vi "_RT_CtrlLoop_ExperimentCondition.vi"(6 "NewExpVar.lvclass":refnum<class "ExpVar.lvclass">, 8 "error in":errorcluster) -> (0 "error out":errorcluster)   [LabVIEW 2018]
uses:
  PublicSubVI/NewExpVar/ExpVar.lvclass
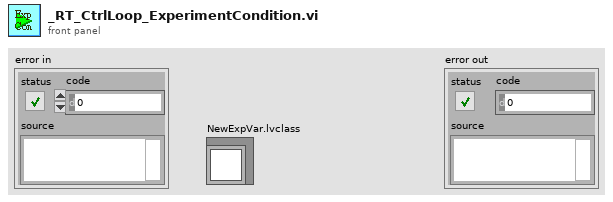
[diagram p1: front panel]
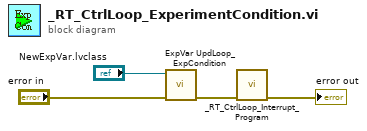
[diagram p0: block diagram]
diagram:
  n1 = call-dynamic "ExpVar UpdLoop_ExpCondition.vi"("error in (no error)"="error in", "NewExpVar in"="NewExpVar.lvclass") -> ("error out"=w2:errorcluster)  [unwired: 8 in, 1 out]
  n2 = call "_RT_CtrlLoop_Interrupt_Program.vi"("error in (no error)"=w2) -> ("error out"=→"error out":errorcluster)  [unwired: 10 in]
